vi "BasicInfo.vi"(8 "error in (no error)":errorcluster, 11 "MGI_MenuItemStatusChange in":refnum<class "MGI_MenuItemStatusChange.lvclass">) -> (0 "error out":errorcluster, 1 "Enabled?":bool, 2 "Checked?":bool, 3 "Tag":string)   [LabVIEW 2016, in "MGI_MenuItemStatusChange.lvclass"]
doc: "Retreives basic information about the last menu click. This VI returns the data of the menu item after the menu click. If you need to view more detailed data or the data before the menu click, use a property node.\n\nAuthored by Derek E. Trepanier\nsupport@mooregoodideas.com\nwww.mooregoodideas.com\n\nCopyright (c) 2012, Moore Good Ideas, Inc.\n\nAll rights reserved.\n\nRedistribution and use in source and binary forms, with or without modification, are permitted provided that the following conditions are met:\n\n * Redistributions of source code must retain the above copyright notice, this list of conditions and the following disclaimer.\n * Redistributions in binary form must reproduce the above copyright notice, this list of conditions and the following disclaimer in the documentation and/or other materials provided with the distribution.\n * Neither the name of Moore Good Ideas, Inc. nor the names of its contributors may be used to endorse or promote products derived from this software without specific prior written permission.\n\nTHIS SOFTWARE IS PROVIDED BY THE COPYRIGHT HOLDERS AND CONTRIBUTORS \"AS IS\" AND ANY EXPRESS OR IMPLIED WARRANTIES, INCLUDING, BUT NOT LIMITED TO, THE IMPLIED WARRANTIES OF MERCHANTABILITY AND FITNESS FOR A PARTICULAR PURPOSE ARE DISCLAIMED. IN NO EVENT SHALL THE COPYRIGHT OWNER OR CONTRIBUTORS BE LIABLE FOR ANY DIRECT, INDIRECT, INCIDENTAL, SPECIAL, EXEMPLARY, OR CONSEQUENTIAL DAMAGES (INCLUDING, BUT NOT LIMITED TO, PROCUREMENT OF SUBSTITUTE GOODS OR SERVICES; LOSS OF USE, DATA, OR PROFITS; OR BUSINESS INTERRUPTION) HOWEVER CAUSED AND ON ANY THEORY OF LIABILITY, WHETHER IN CONTRACT, STRICT LIABILITY, OR TORT (INCLUDING NEGLIGENCE OR OTHERWISE) ARISING IN ANY WAY OUT OF THE USE OF THIS SOFTWARE, EVEN IF ADVISED OF THE POSSIBILITY OF SUCH DAMAGE."
uses:
  <userlib>/_MGI/Menu Building/MenuItemStatusChange/MGI_MenuItemStatusChange.lvclass
  <userlib>/_MGI/Menu Building/MenuItemStatusChange/Read MenuItem.vi
  <userlib>/_MGI/Menu Building/MenuItem/Read Tag.vi
  <userlib>/_MGI/Menu Building/MenuItem/Read Checked.vi
  <userlib>/_MGI/Menu Building/MenuItem/Read Enabled.vi
  <userlib>/_MGI/Menu Building/MenuItem/MGI_MenuItem.lvclass
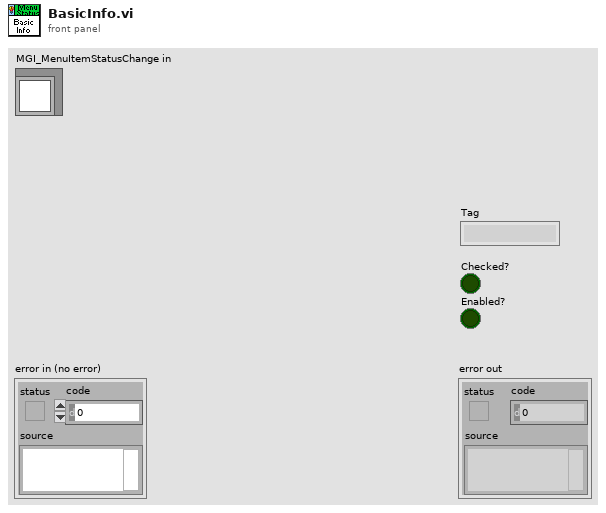
[diagram p1: front panel]
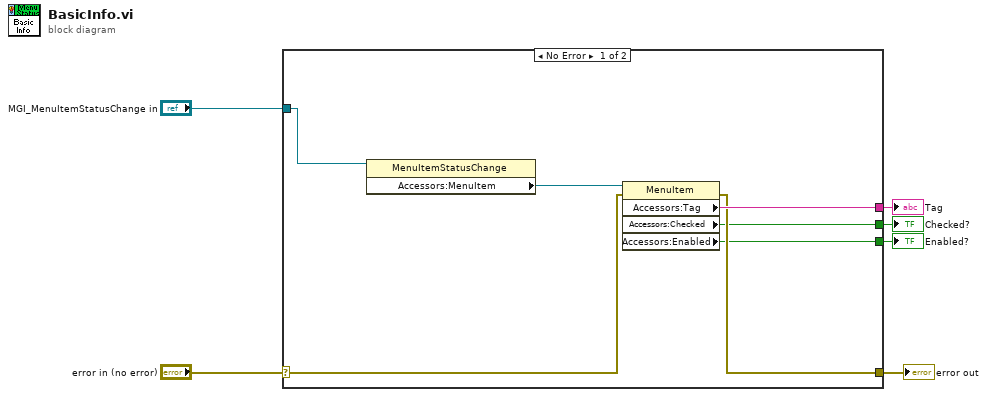
[diagram p0: block diagram]
diagram:
  n1 = case shown="No Error" "error in (no error)" {
    selector: "error in (no error)" -> [w12 w14]
    tunnel: [w11 w14] -> w5
    tunnel: "MGI_MenuItemStatusChange in" -> [w10 _]
    tunnel: [w13 _] -> w3
    tunnel: [w8 _] -> w2
    tunnel: [w7 _] -> w1
    frame No Error {
      n2 = property class="MenuItemStatusChange"(reference=w10) -> ("Accessors:MenuItem"=w9:refnum<data-value>)  [unwired: 1 in, 2 out]
      n3 = property class="MenuItem"(reference=w9, error in=w12) -> (error out=w11:errorcluster, "Accessors:Tag"=w13:string, "Accessors:Checked"=w8:bool, "Accessors:Enabled"=w7:bool)  [unwired: 1 out]
    }
    frame Error {
    }
  }
  "error out" <- w5
  "Tag" <- w3
  "Checked?" <- w2
  "Enabled?" <- w1
